vi "jl-scripts path.vi"() -> ()   [LabVIEW 2018, in "LV-0mq-Julia_roundtrip-lib.lvlib"]
uses:
  LV-0mq-Julia_roundtrip-lib.lvlib
panel:
  out "jl-script file path":path
  out "tmp file path":path
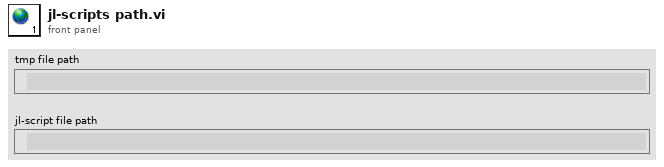
[diagram p1: front panel]
diagram:
